vi "ImplModelFollow_New.vi"(8 "B_Ref":T2, 9 "A_Ref":T2, 10 "B":T2, 11 "A":T2) -> (0 "Error":bool, 3 "IMPLICIT_MODEL_FOLLOWER":T1)   [LabVIEW 2019, in "Trajectory_Library.lvlib"]
doc: "Create implicit model follower\n\nInputs:\n - A < states, states > -- Continuous system matrix of the plant being controlled.\n - B < states, inputs > -- Continuous input matrix of the plant being controlled.\n - A_Ref < states, states > -- Continuous system matrix whose dymanics should be followed.\n - B_Ref < states, inputs > -- Continuous input matrix x whose dymanics should be followed.\n\nOutputs:\n - Error -- If TRUE, an error occured."
uses:
  Trajectory_Library.lvlib
  <vilib>/Analysis/Matrix/Datatypes/RealMatrix.ctl
  IMPLICIT_MODEL_FOLLOWER.ctl
  <vilib>/Analysis/Matrix/Numeric/Subtract/Subtract - RM,RM.vi
  <vilib>/Analysis/7linalg.llb/Solve Linear Equations (multiple right hand).vi
  <vilib>/Analysis/Matrix/Numeric/Multiply/Multiply - RM,R.vi
  <vilib>/Analysis/Matrix/NI_Matrix.lvlib
  <vilib>/Analysis/NI_AALPro.lvlib
panel:
  # "<states, states>"
  # "<states, inputs>"
  # "<states, states>"
  # "<states, inputs>"
  # "<States,States>"
  # "<States,Inputs>"
  # "<Inputs,1>"
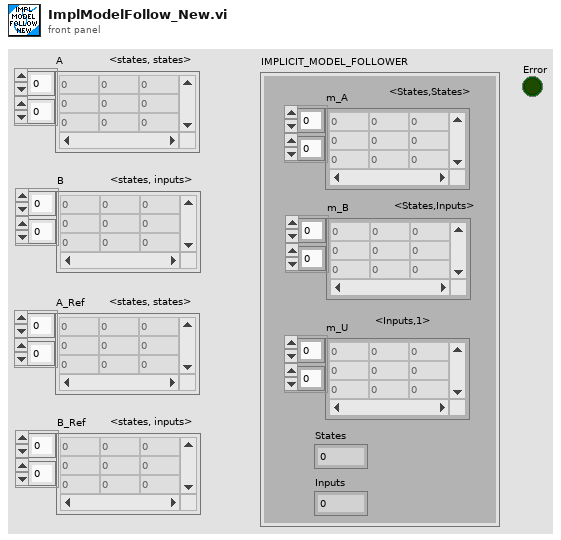
[diagram p1: front panel]
types:
  T1 = typedef "Trajectory_Library.lvlib/IMPLICIT_MODEL_FOLLOWER.ctl" = cluster{"m_A":T2, "m_B":T2, "m_U":T2, "States":i32, "Inputs":i32}
  T2 = typedef "NI_Matrix.lvlib/RealMatrix.ctl" = dbl[][]
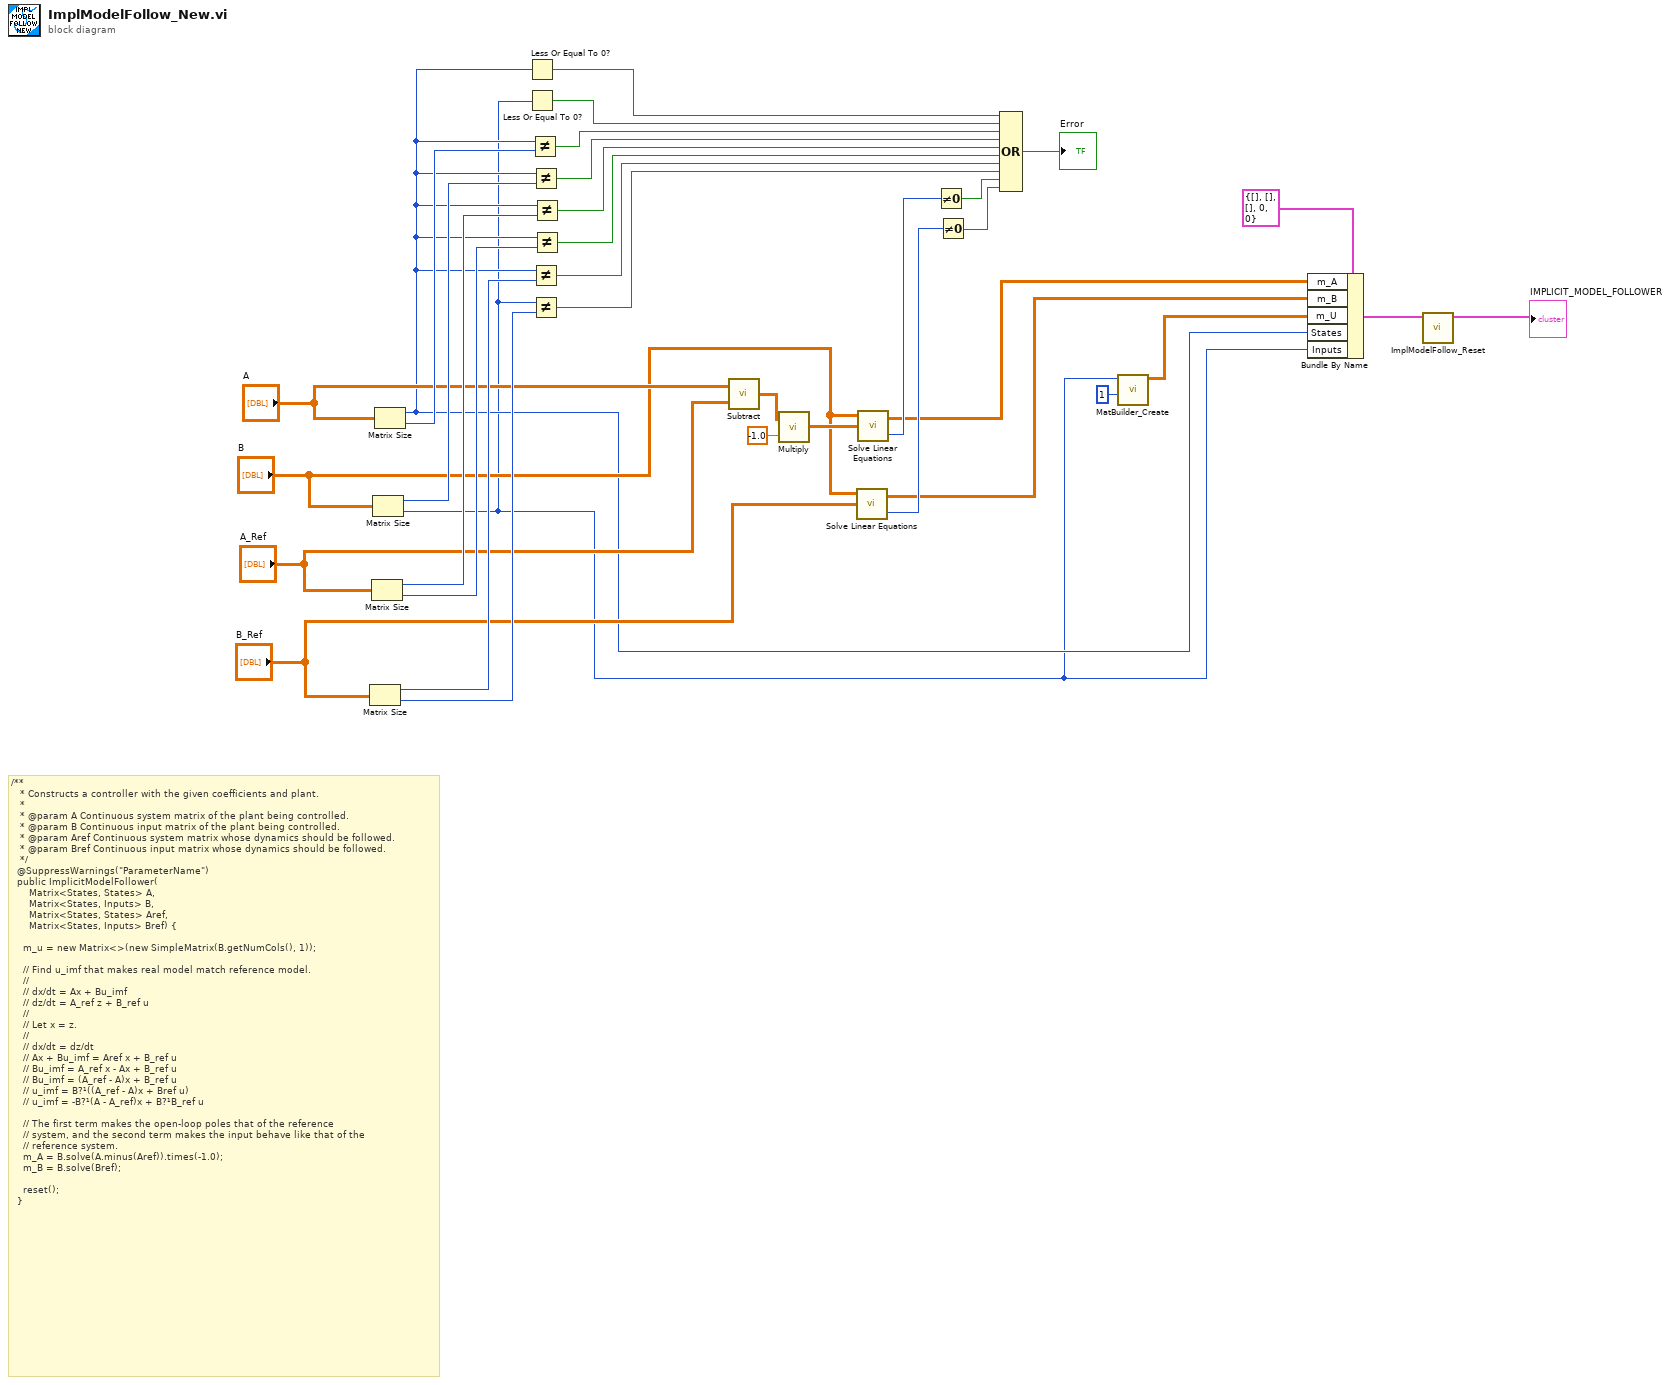
[diagram p0: block diagram]
diagram:
  # "/**\n   * Constructs a controller with the given coefficients and plant.\n   *\n   * @param A Continuous system matrix of the plant being controlled.\n   * @param B Continuous input matrix of the plant being controlled.\n   * @param Aref Continuous system matrix whose dynamics should be followed.\n   * @param Bref Continuous input matrix whose dynamics should be followed.\n   */\n  @SuppressWarnings(\"ParameterName\")\n  public ImplicitModelFollower(\n      Matrix<States, States> A,\n      Matrix<States, Inputs> B,\n      Matrix<States, States> Aref,\n      Matrix<States, Inputs> Bref) {\n\n    m_u = new Matrix<>(new SimpleMatrix(B.getNumCols(), 1));\n\n    // Find u_imf that makes real model match reference model.\n    //\n    // dx/dt = Ax + Bu_imf\n    // dz/dt = A_ref z + B_ref u\n    //\n    // Let x = z.\n    //\n    // dx/dt = dz/dt\n    // Ax + Bu_imf = Aref x + B_ref u\n    // Bu_imf = A_ref x - Ax + B_ref u\n    // Bu_imf = (A_ref - A)x + B_ref u\n    // u_imf = B?¹((A_ref - A)x + Bref u)\n    // u_imf = -B?¹(A - A_ref)x + B?¹B_ref u\n\n    // The first term makes the open-loop poles that of the reference\n    // system, and the second term makes the input behave like that of the\n    // reference system.\n    m_A = B.solve(A.minus(Aref)).times(-1.0);\n    m_B = B.solve(Bref);\n\n    reset();\n  }"
  n1 = Matrix Size(0:"B_Ref") -> (1:w31:i32, 2:w30:i32)
  n2 = Matrix Size(0:"A_Ref") -> (1:w33:i32, 2:w32:i32)
  n3 = Matrix Size(0:"B") -> (1:w34:i32, 2:w5:i32)
  n4 = Matrix Size(0:"A") -> (1:w8:i32, 2:w35:i32)
  n5 = Less Or Equal To 0?(x=w8) -> (x <= 0?=w7:bool)
  n6 = Less Or Equal To 0?(x=w5) -> (x <= 0?=w6:bool)
  n7 = Not Equal?(x=w8, y=w35) -> (x != y?=w29:bool)
  n8 = Not Equal?(x=w8, y=w34) -> (x != y?=w27:bool)
  n9 = Not Equal?(x=w8, y=w31) -> (x != y?=w24:bool)
  n10 = Not Equal?(x=w5, y=w30) -> (x != y?=w23:bool)
  n11 = Not Equal?(x=w8, y=w33) -> (x != y?=w26:bool)
  n12 = Not Equal?(x=w8, y=w32) -> (x != y?=w25:bool)
  n13 = call-poly <vilib>:"Subtract.vi"("Real Matrix B"="A_Ref", "Real Matrix A"="A") -> ("A - B"=w19:T2)
  n14 = call-poly <vilib>:"Multiply.vi"("Real Scalar c"=-1.0 ("y"), "Real Matrix A"=w19) -> ("A * c"=w18:T2)
  n15 = call-poly <vilib>:"Solve Linear Equations.vi"("Known Matrix"="B_Ref", "Input Matrix"="B") -> ("error"=w13:i32, "Solution Matrix"=w9:T2)  [unwired: 1 in]
  n16 = call-poly <vilib>:"Solve Linear Equations.vi"("Known Matrix"=w18, "Input Matrix"="B") -> ("error"=w12:i32, "Solution Matrix"=w10:T2)  [unwired: 1 in]
  n17 = Not Equal To 0?(x=w12) -> (x != 0?=w15:bool)
  n18 = Not Equal To 0?(x=w13) -> (x != 0?=w14:bool)
  n19 = Compound Arithmetic op=OR(w7, w6, w29, w27, w26, w25, w24, w23, w15, w14) -> (→"Error":bool)
  n20 = call "MatBuilder_Create.vi"("Columns"=1, "Rows"=w5) -> ("output matrix"=w3:T2)  [unwired: 9 in]
  n21 = Bundle By Name(cluster=T1 {"m_A"=[], "m_B"=[], "m_U"=[], "States"=0, "Inputs"=0} ("IMPLICIT_MODEL_FOLLOWER"), "m_A"=w10, "m_B"=w9, "m_U"=w3, "States"=w8, "Inputs"=w5) -> (w2:T1)
  n22 = call "ImplModelFollow_Reset.vi"("in IMPLICIT_MODEL_FOLLOWER"=w2) -> ("out IMPLICIT_MODEL_FOLLOWER"=→"IMPLICIT_MODEL_FOLLOWER":T1)  [unwired: 10 in]
